vi "F Dwf Analog In Sampling Slope Get.vi"(8 "error in (no error)":errorcluster, 10 "pslope":i32, 11 "hdwf":i32) -> (0 "error out":errorcluster, 2 "pslope out":i32, 3 "function return":i32)   [LabVIEW 2021, in "Olasdwf.lvlib"]
doc: "DWFAPI int FDwfAnalogInSamplingSlopeGet(HDWF hdwf, DwfTriggerSlope *pslope);"
uses:
  Olasdwf.lvlib
  Windows/System32/dwf.dll
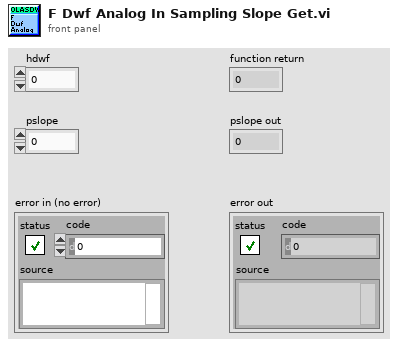
[diagram p1: front panel]
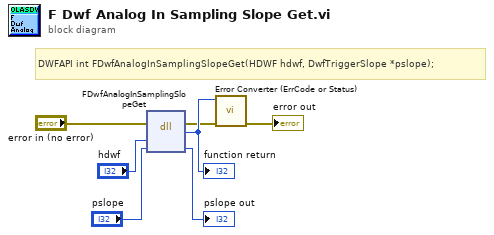
[diagram p0: block diagram]
diagram:
  # "DWFAPI int FDwfAnalogInSamplingSlopeGet(HDWF hdwf, DwfTriggerSlope *pslope);"
  n1 = dll-call lib="/Windows/System32/dwf.*" fn="FDwfAnalogInSamplingSlopeGet"(error in="error in (no error)", "hdwf"="hdwf", "pslope"="pslope") -> (error out=w2:errorcluster, w7:i32, "pslope"=→"pslope out":i32)  [unwired: 3 in, 1 out]
  "function return" <- w7
  n2 = call "Error Converter (ErrCode or Status).vi"("error in (no error)"=w2, "error code"=w7) -> ("error out"=→"error out":errorcluster)  [unwired: 9 in]
